vi "SVT Human Vibration Weighting Filter (octave).vi"   [LabVIEW 2017, in "SoundVib_Octave_2014 standard.lvlib"]
doc: "Applies the selected human vibration weighting to octave spectra. This VI weights each spectral bin according to the attenuation of the specified filter at the bin center frequency. You can use this VI in a loop to process multiple blocks. Wire data to the <B>octave spectrum</B> input to determine the polymorphic instance to use or manually select the instance."
uses:
  <vilib>/addons/Sound and Vibration/svt_Octave/SoundVib_Octave_2014 standard.lvlib
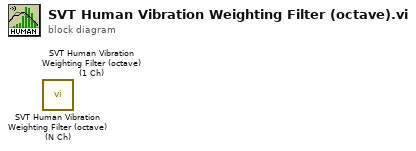
[diagram p0: block diagram]
diagram:
  n1 = call <vilib>:"SVT Human Vibration Weighting Filter (octave) (N Ch).vi"() -> ()  [unwired: 11 in, 5 out]
  n2 = call <vilib>:"SVT Human Vibration Weighting Filter (octave) (1 Ch).vi"() -> ()  [unwired: 11 in, 5 out]
